vi "CPU_MEM_RAM_RE_All.vi"() -> (2 "mem":u8[](array[numeric]))   [LabVIEW 2018]
uses:
  CPU_MEM_references.vi
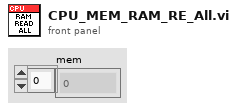
[diagram p1: front panel]
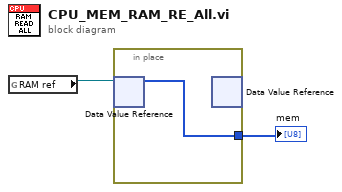
[diagram p0: block diagram]
diagram:
  n1 = global read "CPU_MEM_references.vi" "RAM ref"() -> (w2:refnum<data-value>)
  n2 = in-place {
    in-place-border: [w3] -> w1
    n3 = in-place-dvr #1(w2) -> (w3:u8[])  [unwired: 1 out]
    n4 = in-place-dvr #1() -> ()  [unwired: 1 in, 2 out]
  }
  "mem" <- w1
